vi "RT Streams Config.vi"() -> ()   [LabVIEW 2014]
panel:
  in  "RT writer name":refnum<k21>
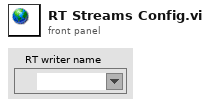
[diagram p1: front panel]
diagram:
